vi "0,360 to -180,180.vi"(11 "Input [0,360]":dbl) -> (3 "Output [-180,180]":dbl)   [LabVIEW 2015]
doc: "Converts an angle from the range [0,360] to the range [-180,180]."
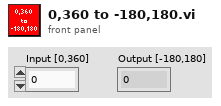
[diagram p1: front panel]
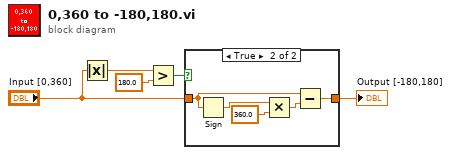
[diagram p0: block diagram]
diagram:
  n1 = Absolute Value(x="Input [0,360]") -> (abs(x)=w1:dbl)
  n2 = Greater?(x=w1, y=180.0) -> (0:w4:bool)
  n3 = case shown="True" w4 {
    tunnel: "Input [0,360]" -> [w6 w11]
    tunnel: [w6 w7] -> w2
    frame False {
    }
    frame True {
      n4 = Sign(1:w11) -> (0:w10:dbl)
      n5 = Multiply(x=w10, y=360.0) -> (x*y=w8:dbl)
      n6 = Subtract(x=w11, y=w8) -> (x-y=w7:dbl)
    }
  }
  "Output [-180,180]" <- w2
